vi "GPIB Device.vi"(0 "Point #":i32) -> (1 "GPIB Data Out":dbl[](array[numeric]) format="%.2e", 2 "Stop Out":bool)   [LabVIEW 2021]
doc: "VI which calls the appropriate GPIB routines for a variety of instruments.\nScott Hannahs, NHMFL-FSU, Nov. 1993"
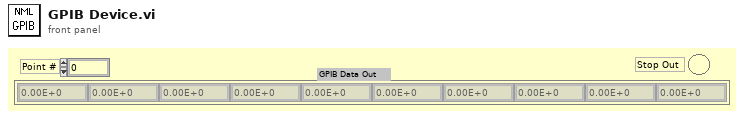
[diagram p1: front panel]
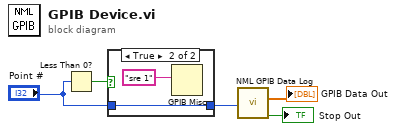
[diagram p0: block diagram]
diagram:
  n1 = Less Than 0?(x="Point #") -> (x < 0?=w3:bool)
  n2 = case shown="True" w3 {
    tunnel: [w6 w7] -> w1
    tunnel: "Point #" -> [w6 w7]
    frame False {
    }
    frame True {
      n3 = GPIB Misc(0:"sre 1") -> ()  [unwired: 1 in, 3 out]
    }
  }
  n4 = call "NML GPIB Data Log.vi"("Point #"=w1) -> ("GPIB Data"=→"GPIB Data Out":dbl[], "Stop"=→"Stop Out":bool)
